vi "SP - set value BOOL.vi"(8 "error in (no error)":errorcluster, 11 "JSON string":string) -> (0 "error out":errorcluster, 3 "value":string)   [LabVIEW 2020, in "ui-testing.lvlib"]
doc: "copyright: Thomas Zilliox©"
uses:
  ui-testing.lvlib
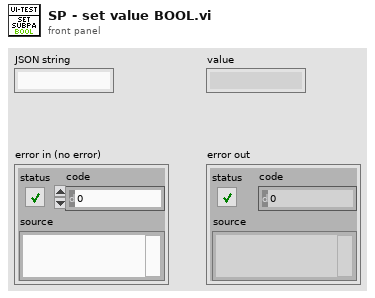
[diagram p1: front panel]
types:
  T1 = cluster{"subpanel":string, "control":string, "value":bool}
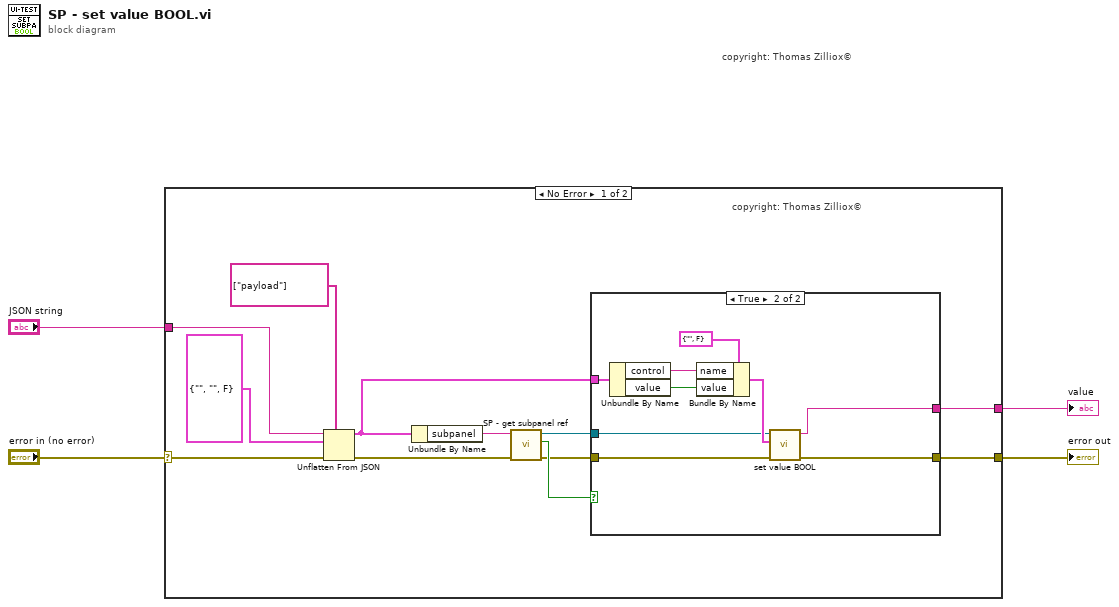
[diagram p0: block diagram]
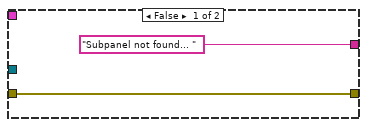
[diagram p2: hidden frame]
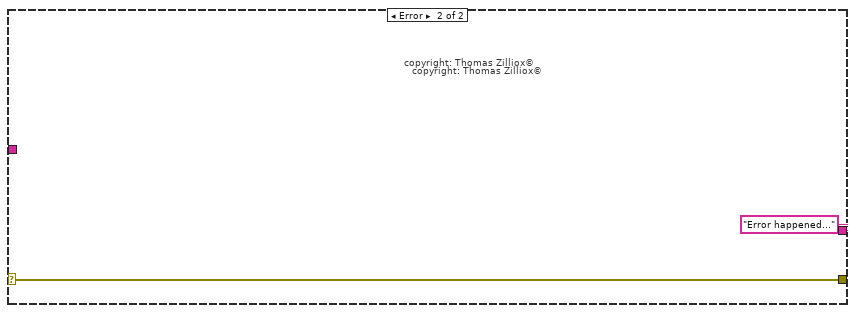
[diagram p3: hidden frame]
diagram:
  # "copyright: Thomas Zilliox©"
  n1 = case shown="No Error" "error in (no error)" {
    selector: "error in (no error)" -> [w13 w29]
    tunnel: "JSON string" -> [w15 _]
    tunnel: [w14 w29] -> w3
    tunnel: [w11 "Error happened..."] -> w1
    frame No Error {
      # "copyright: Thomas Zilliox©"
      n2 = Unflatten From JSON(path=string[] ["payload"], JSON string=w15, type and defaults=T1 {"subpanel"="", "control"="", "value"=FALSE}, error in (no error)=w13) -> (value=w9:T1, error out=w8:errorcluster)  [unwired: 3 in]
      n3 = Unbundle By Name(w9) -> ("subpanel"=w10:string)
      n4 = call "SP - get subpanel ref.vi"("error in (no error)"=w8, "subpanel"=w10) -> ("error out"=w5:errorcluster, "subpanel found ?"=w6:bool, "subpanel VI ref"=w7:refnum<vi>)  [unwired: 6 in, 1 out]
      n5 = case shown="True" w6 {
        tunnel: [w18 w26] -> w14
        tunnel: w5 -> [w18 w25]
        tunnel: ["Subpanel not found... " ("result string") w27] -> w11
        tunnel: w9 -> [_ w22]
        tunnel: w7 -> [_ w19]
        frame False {
        }
        frame True {
          n6 = Unbundle By Name(w22) -> ("control"=w20:string, "value"=w21:bool)
          n7 = Bundle By Name(cluster=cluster{"name":string, "value":bool} {"name"="", "value"=FALSE} ("Payload"), "name"=w20, "value"=w21) -> (w23:cluster{"name":string, "value":bool})
          n8 = call "set value BOOL.vi"("error in (no error)"=w25, "Payload"=w23, "VI Ref"=w19) -> ("error out"=w26:errorcluster, "return value"=w27:string)  [unwired: 7 in]
        }
      }
    }
    frame Error {
      # "copyright: Thomas Zilliox©"
      # "copyright: Thomas Zilliox©"
    }
  }
  "error out" <- w3
  "value" <- w1
